vi "working_interface.vi"(10 "VISA resource name":refnum<visa-resource-name>="TRIG") -> (2 "data in delay generator (s)":dbl[](array[numeric]) caption="delay array" min=0.0 max=2000.0 format="%.3f")   [LabVIEW 2011]
panel:
  in  "time unit":enum16{"s", "ms", "us", "ns"}(ring)=enum."us"
  in  "resolution":i32=100
  in  "duration array":dbl[](array[numeric]) format="%.3f"
  in  "start time array":dbl[](array[numeric]) format="%.3f"
  out "Digital Waveform Graph":digitalwaveform(graph)
  in  "trigger":bool
  in  "write data":bool
  in  "read delay data":bool
  in  "stop":bool
  # "timing values are only relative,\n the absolute values are given in the\ndelay array!!!\n\nt0 and t can not be written to the device, t0 is always 0\nand  t is always the longest time + 25ns. However, t is \nused to display how long the nozzle is open to give a real \nrepresentation in the diagram (and only there). \nYou can change that time to pretty much any value, \nbut the nozzle itself is not controlled through the labview\n software. You have to set the time manually at the \nnozzle driver and ideally you should then enter that time\nfor t as well!\n\ndelay array index:\n0 - t0 = nozzle start (TTL) = 0\n1 - nozzle duration\n2 - power AMP START\n3 - power AMP STOP\n4 - AWG START (TTL)\n5 - AWG STOP (NA)\n6 - SWITCH ON \n7 - SWITCH OFF\n8 - OSC START (TTL)\n9 - OSC STOP (NA)\n\nTTL -> tool starts on rising flank\nof signal, hence the falling flank \nand the duration are not important!"
  # "delay array index:\n0 - to = nozzle start (TTL) = 0\n1 - t = nozzle duration\n2 - A = power AMP START\n3 - B = power AMP STOP\n4 - C = AWG START (TTL)\n5 - D = AWG STOP (NA)\n6 - E = SWITCH ON \n7 - F = SWITCH OFF\n8 - G = OSC START (TTL)\n9 - H = OSC STOP (NA)\n\nTTL -> tool starts on rising flank\nof signal, hence the falling flank \nand the duration are not important!"
  # "t0 is always 0"
  # "AWG must start after power AMP is on \nand while it is still on!"
  # "SWITCH must NOT switch ON before \npower AMP is off!"
  # "t0"
  # "t"
  # "A"
  # "B"
  # "C"
  # "D"
  # "E"
  # "F"
  # "G"
  # "H"
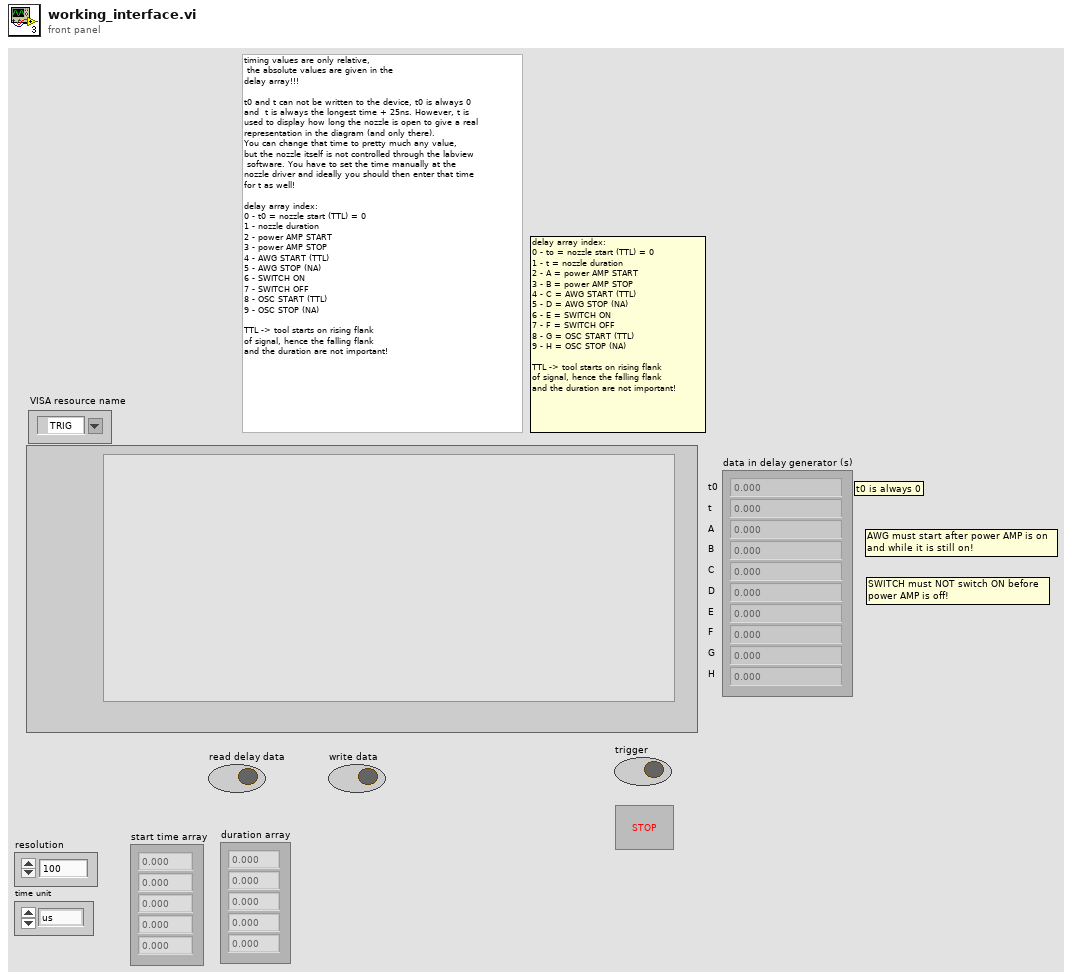
[diagram p1: front panel]
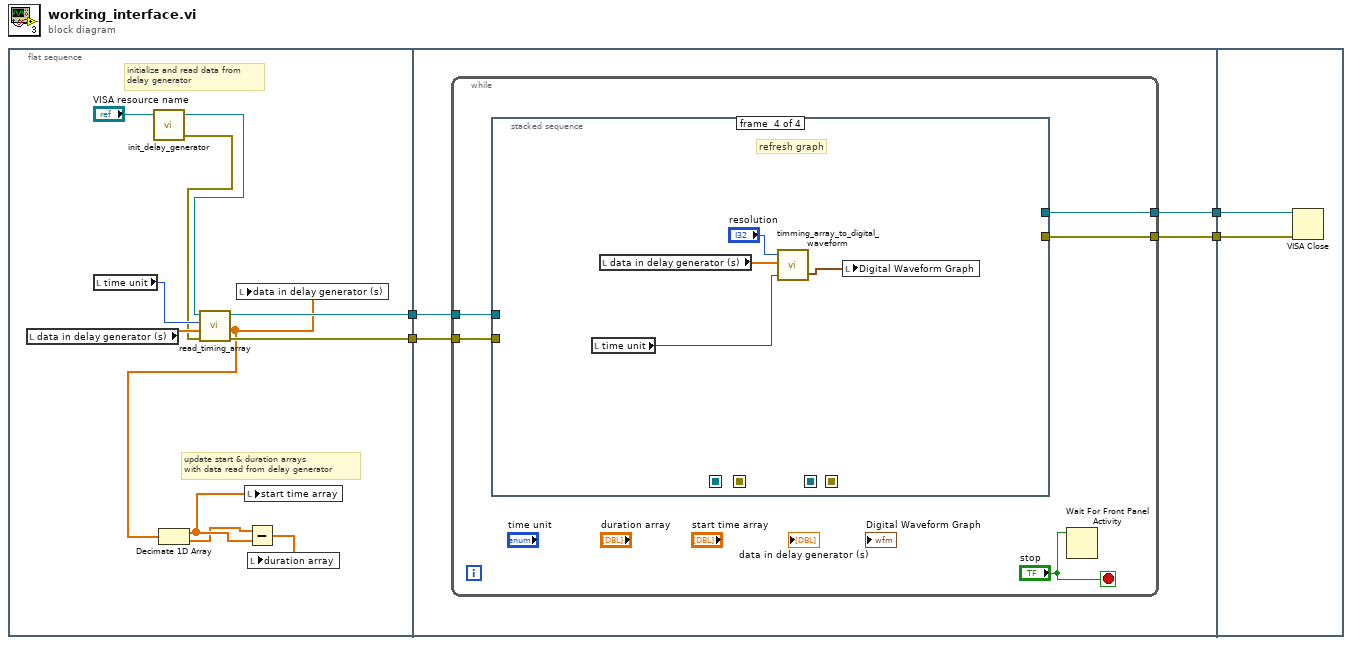
[diagram p0: block diagram]
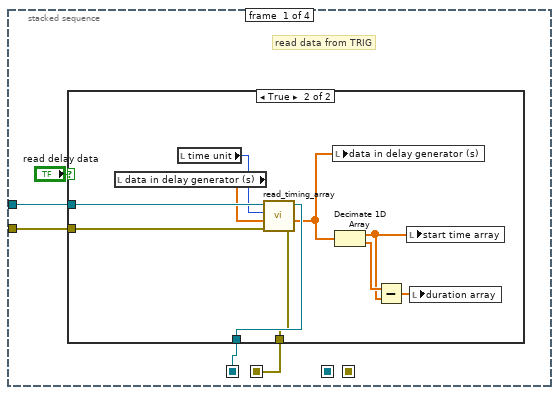
[diagram p2: hidden frame]
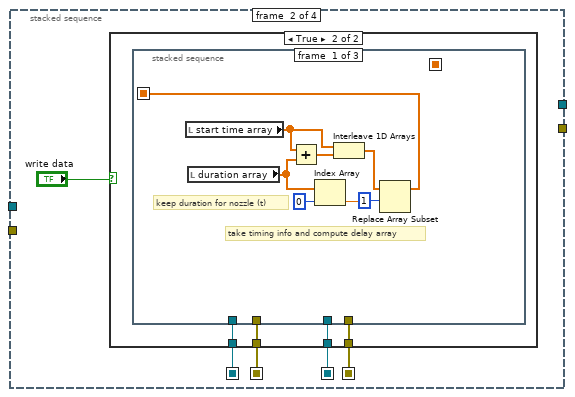
[diagram p4: hidden frame]
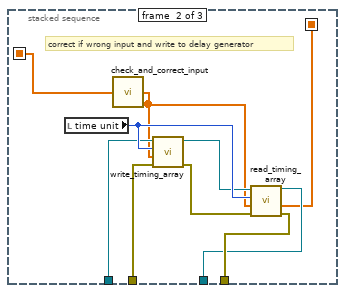
[diagram p6: hidden frame]
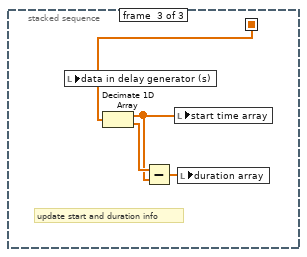
[diagram p7: hidden frame]
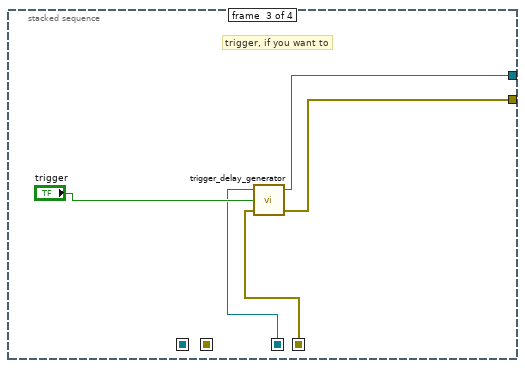
[diagram p8: hidden frame]
diagram:
  n1 = flat-sequence {
    tunnel: [w13] -> w4
    tunnel: [w14] -> w3
    tunnel: w4 -> [w19]
    tunnel: w3 -> [w18]
    tunnel: [w17] -> w2
    tunnel: [w16] -> w1
    tunnel: w2 -> [w85]
    tunnel: w1 -> [w84]
    frame #0 {
      # "update start & duration arrays \nwith data read from delay generator"
      # "initialize and read data from \ndelay generator"
      n2 = local read "data in delay generator (s)"() -> (w15:dbl[])
      n3 = local read "time unit"() -> (w9:enum16{"s", "ms", "us", "ns"})
      n4 = call "init_delay_generator.vi"("VISA resource name"="VISA resource name") -> ("error out"=w5:errorcluster, "VISA resource name out"=w6:refnum<visa-resource-name>)  [unwired: 3 in]
      n5 = call "read_timing_array.vi"("error in"=w5, "input array"=w15, "time unit"=w9, "VISA resource in"=w6) -> ("error out 2"=w14:errorcluster, "delay array"=w8:dbl[], "VISA resource out"=w13:refnum<visa-resource-name>)  [unwired: 1 in]
      n6 = Decimate 1D Array(w8) -> (w11:dbl[], w10:dbl[])
      n7 = local write "data in delay generator (s)"(w8) -> ()
      n8 = local write "start time array"(w11) -> ()
      n9 = Subtract(x=w10, y=w11) -> (x-y=w12:dbl[])
      n10 = local write "duration array"(w12) -> ()
    }
    frame #1 {
      n11 = while {
        tunnel: w18 -> [w22]
        tunnel: [w24] -> w17
        tunnel: [w23] -> w16
        tunnel: w19 -> [w20]
        stop <- "stop" stop-if-true
        n12 = stacked-sequence {
          seq-local: [w27 _ _ _] -> [_ w43 _ _]
          seq-local: [w26 _ _ _] -> [_ w42 _ _]
          seq-local: [_ w45 _ _] -> [_ _ w76 _]
          seq-local: [_ w44 _ _] -> [_ _ w77 _]
          tunnel: w20 -> [w29 _ _ _]
          tunnel: w22 -> [w28 _ _ _]
          tunnel: [_ _ w75 _] -> w23
          tunnel: [_ _ w79 _] -> w24
          frame #0 {
            # "read data from TRIG"
            n13 = case shown="True" "read delay data" {
              tunnel: w29 -> [w30 w41]
              tunnel: w28 -> [w31 w40]
              tunnel: [w30 w39] -> w27
              tunnel: [w31 w38] -> w26
              frame False {
              }
              frame True {
                n14 = local read "data in delay generator (s)"() -> (w37:dbl[])
                n15 = local read "time unit"() -> (w36:enum16{"s", "ms", "us", "ns"})
                n16 = call "read_timing_array.vi"("error in"=w40, "input array"=w37, "time unit"=w36, "VISA resource in"=w41) -> ("error out 2"=w38:errorcluster, "delay array"=w33:dbl[], "VISA resource out"=w39:refnum<visa-resource-name>)  [unwired: 1 in]
                n17 = local write "data in delay generator (s)"(w33) -> ()
                n18 = Decimate 1D Array(w33) -> (w32:dbl[], w34:dbl[])
                n19 = Subtract(x=w34, y=w32) -> (x-y=w35:dbl[])
                n20 = local write "start time array"(w32) -> ()
                n21 = local write "duration array"(w35) -> ()
              }
            }
          }
          frame #1 {
            n22 = case shown="True" "write data" {
              tunnel: [w48 w49] -> w45
              tunnel: [w47 w52] -> w44
              tunnel: w43 -> [w48 w51]
              tunnel: w42 -> [w47 w50]
              frame False {
              }
              frame True {
                n23 = stacked-sequence {
                  seq-local: [w53 _ _] -> [_ w62 _]
                  seq-local: [_ w61 _] -> [_ _ w72]
                  tunnel: [_ w70 _] -> w52
                  tunnel: w51 -> [_ w68 _]
                  tunnel: w50 -> [_ w67 _]
                  tunnel: [_ w64 _] -> w49
                  frame #0 {
                    # "take timing info and compute delay array"
                    # "keep duration for nozzle (t)"
                    n24 = local read "start time array"() -> (w59:dbl[])
                    n25 = local read "duration array"() -> (w58:dbl[])
                    n26 = Add(x=w59, y=w58) -> (x+y=w60:dbl[])
                    n27 = Index Array(array=w58, index=0) -> (element=w54:dbl)
                    n28 = Interleave 1D Arrays(w59, w60) -> (w56:dbl[])
                    n29 = Replace Array Subset(array=w56, new element=w54, index=1) -> (w53:dbl[])
                  }
                  frame #1 {
                    # "correct if wrong input and write to delay generator"
                    n30 = local read "time unit"() -> (w69:enum16{"s", "ms", "us", "ns"})
                    n31 = call "check_and_correct_input.vi"("delay array"=w62) -> ("corrrected delay array"=w63:dbl[])  [unwired: 4 in]
                    n32 = call "write_timing_array.vi"("error in"=w67, "delay array"=w63, "time unit"=w69, "VISA resource in"=w68) -> ("error out 2"=w65:errorcluster, "VISA resource out"=w66:refnum<visa-resource-name>)  [unwired: 2 in]
                    n33 = call "read_timing_array.vi"("error in"=w65, "input array"=w63, "time unit"=w69, "VISA resource in"=w66) -> ("error out 2"=w70:errorcluster, "delay array"=w61:dbl[], "VISA resource out"=w64:refnum<visa-resource-name>)  [unwired: 1 in]
                  }
                  frame #2 {
                    # "update start and duration info"
                    n34 = local write "data in delay generator (s)"(w72) -> ()
                    n35 = Decimate 1D Array(w72) -> (w71:dbl[], w74:dbl[])
                    n36 = Subtract(x=w74, y=w71) -> (x-y=w73:dbl[])
                    n37 = local write "start time array"(w71) -> ()
                    n38 = local write "duration array"(w73) -> ()
                  }
                }
              }
            }
          }
          frame #2 {
            # "trigger, if you want to"
            n39 = call "trigger_delay_generator.vi"("error in (no error)"=w77, "Boolean"="trigger", "VISA resource name"=w76) -> ("error out"=w75:errorcluster, "VISA resource name 2"=w79:refnum<visa-resource-name>)  [unwired: 1 in]
          }
          frame #3 {
            # "refresh graph"
            n40 = local read "time unit"() -> (w80:enum16{"s", "ms", "us", "ns"})
            n41 = local read "data in delay generator (s)"() -> (w83:dbl[])
            n42 = call "timming_array_to_digital_waveform.vi"("time unit"=w80, "delay array"=w83, "resolution"="resolution") -> ("digital waveform"=w82:digitalwaveform)  [unwired: 1 in]
            n43 = local write "Digital Waveform Graph"(w82) -> ()
          }
        }
        n44 = Wait For Front Panel Activity(3:"stop") -> ()  [unwired: 2 in, 1 out]
      }
    }
    frame #2 {
      n45 = VISA Close(VISA resource name=w85, error in (no error)=w84) -> ()  [unwired: 1 out]
    }
  }
